vi "2 ‚crans.vi"() -> ()   [LabVIEW 2013]
uses:
  <vilib>/Instr/_visa.llb/VISA Configure Serial Port (Instr).vi
panel:
  out "Distance du drone à la caméra":dbl format="%#_4g"
  out "Taille 2":u32
  out "Taille 1":u32
  out "Taille 4":u32
  out "Taille 3":u32
  out "Y3":u32
  out "X3":u32
  out "Y":u32
  out "X":u32
  out "Y":u32
  out "X1":u32
  out "Y":u32
  out "X":u32
  in  "Y max":i32
  in  "X max":i32
  in  "Y min":i32
  in  "X min":i32
  out "new picture en sortie 2":picture caption="Camera 2"
  out "Chaîne":string
  in  "Attente (ms)":u32=80
  out "new picture en sortie":picture caption="Camera 1"
  out "Chaîne vide":bool
  out "Intrusion dans la\nzone de sécurité !":bool
  out "bytes read":u32
  in  "Source":refnum<visa-resource-name>="COM1"
  in  "stop":bool
  in  "Play":bool
  in  "path to BMP file":path
  # "Ce programme est conçu pour repérer la position des quatre drones ou moins dans une zone a surveiller.\n\nLorsque que l'un des drones rentre dans la zone de haute sécurité ( zone grisée ) une alarme se déclanche, \nen effet, la LED est verte si aucun drone n'est repéré dans la cette zone et elle est rouge si un drone est\ndétecté.\n\nLe programme nous donne aussi la position des drones. Ces informations sont transmises via Wi-Fi grâce à un module X-Bee connecté a un port USB."
  # "La LED de couleur verte indique que les\ndonnées sont en cours de traitement. \nLa LED de couleur rouge indique que le \nprogramme attend les données."
  # "ATTENTION !\nVeillez à ce que la souce de donnée soit\nbranchée sur le port ci-contre.\nSi le port USB correspondant ne s'affiche\npas cliquez sur Rafraichir puis sélectionner \nbon port."
  # "Ce voyant reste vert quand aucun drone ne se trouve dans la zone de sécurité.\nCe voyant s'allume en rouge lorsqu'un drone rentre dans la zone de sécurité.\n\nUn signal sonore est également émis lorsqu'un drone entre dans la zone."
  # "Play / Pause"
  # "Arrêter le programme"
  # "Coordonnées de\nla zone de sécurité"
  # "drone violet"
  # "drone violet"
  # "Position"
  # "Position"
  # "Taille"
  # "Taille"
  # "drone jaune"
  # "drone jaune"
  # "Position"
  # "Position"
  # "Taille"
  # "Taille"
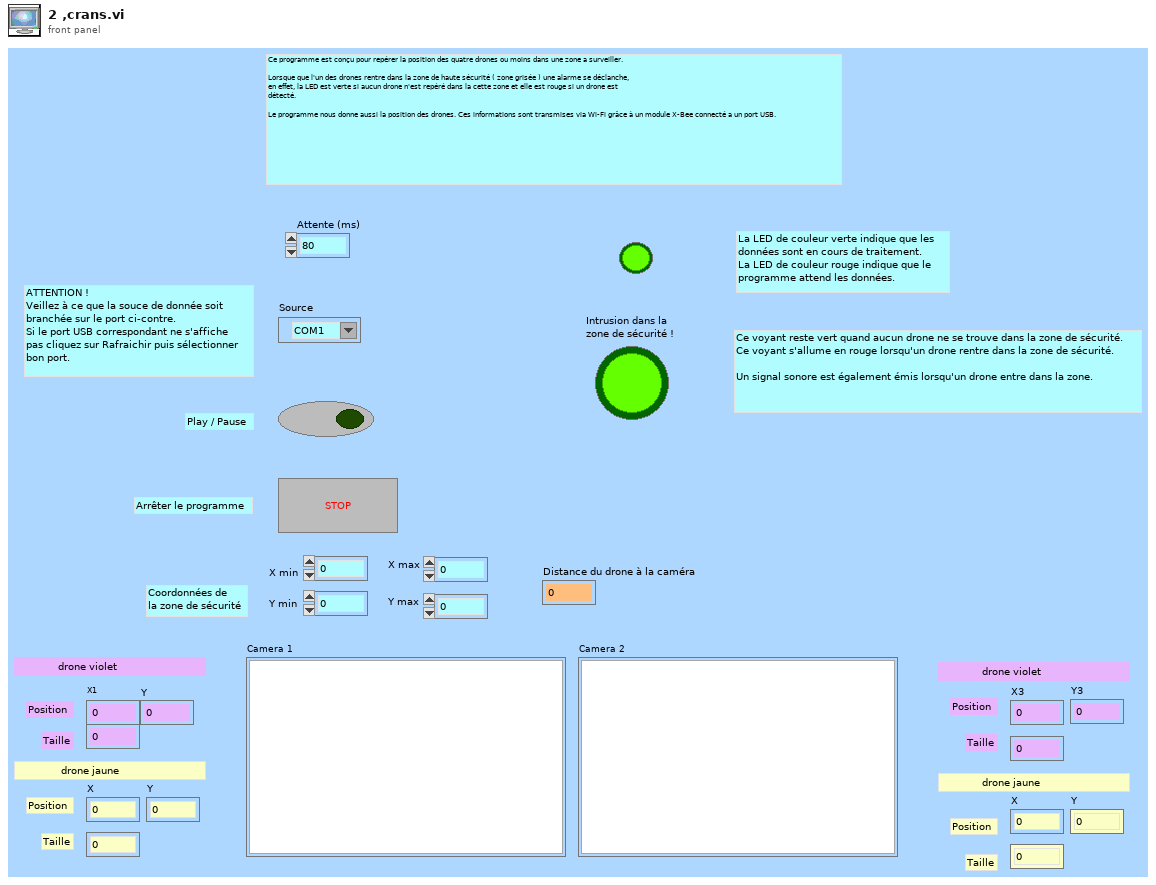
[diagram p1: front panel]
types:
  T1 = typedef "imagedata.ctl" = cluster{"image type":i32, "image depth":i32, "image":u8[], "mask":u8[], "colors":u32[], "Rectangle":cluster{"left":i16, "top":i16, "right":i16, "bottom":i16}}
  T2 = enum32{"Solid", "Dash", "Dot", "DashDot", "DashDotDot"}
  T3 = cluster{cluster{u32, cluster{u32, u32}}, cluster{u32, cluster{u32, u32}}, cluster{u32, cluster{u32, u32}}, cluster{u32, cluster{u32, u32}}}
  T4 = cluster{"S1":cluster{"X (S2;b1) ":u32, "Y (S2;b1)":u32}, "S2":cluster{"X (S2;b1) ":u32, "Y (S2;b1)":u32}, "S3":cluster{"X (S2;b1) ":u32, "Y (S2;b1)":u32}, "S4":cluster{"X (S2;b1) ":u32, "Y (S2;b1)":u32}, "taille (S1)":u32, "taille (S2)":u32, "taille (S3)":u32, "taille (S4)":u32}
  T5 = cluster{cluster{"taille (S1)":u32, "S1":cluster{"X (S2;b1) ":u32, "Y (S2;b1)":u32}}, cluster{"taille (S2)":u32, "S2":cluster{"X (S2;b1) ":u32, "Y (S2;b1)":u32}}, cluster{"taille (S3)":u32, "S3":cluster{"X (S2;b1) ":u32, "Y (S2;b1)":u32}}, cluster{"taille (S4)":u32, "S4":cluster{"X (S2;b1) ":u32, "Y (S2;b1)":u32}}}
  T6 = cluster{"S1":cluster{"X (S1;b1)":u32, "Y (S1;b1)":u32}, "S2":cluster{"X (S1;b2) ":u32, "Y (S1;b2)":u32}, "S3":cluster{"X (S2;b1) ":u32, "Y (S2;b1)":u32}, "S4":cluster{"X (S2;b2)":u32, "Y (S2;b2)":u32}}
  T7 = cluster{"X min":i32, "Y min":i32, "X max":i32, "Y max":i32}
  T8 = cluster{"taille (S1)":u32, "Style":enum32{"Solid", "Dash", "Dot", "DashDot", "DashDotDot"}}
  T9 = cluster{"taille (S3)":u32, "Style":enum32{"Solid", "Dash", "Dot", "DashDot", "DashDotDot"}}
  T10 = cluster{"taille (S4)":u32, "Style":enum32{"Solid", "Dash", "Dot", "DashDot", "DashDotDot"}}
  T11 = cluster{"taille (S2)":u32, "Style":enum32{"Solid", "Dash", "Dot", "DashDot", "DashDotDot"}}
  T12 = cluster{"taille (S1)":u32, "S1":cluster{"X (S2;b1) ":u32, "Y (S2;b1)":u32}}
  T13 = cluster{"taille (S2)":u32, "S2":cluster{"X (S2;b1) ":u32, "Y (S2;b1)":u32}}
  T14 = cluster{"taille (S3)":u32, "S3":cluster{"X (S2;b1) ":u32, "Y (S2;b1)":u32}}
  T15 = cluster{"taille (S4)":u32, "S4":cluster{"X (S2;b1) ":u32, "Y (S2;b1)":u32}}
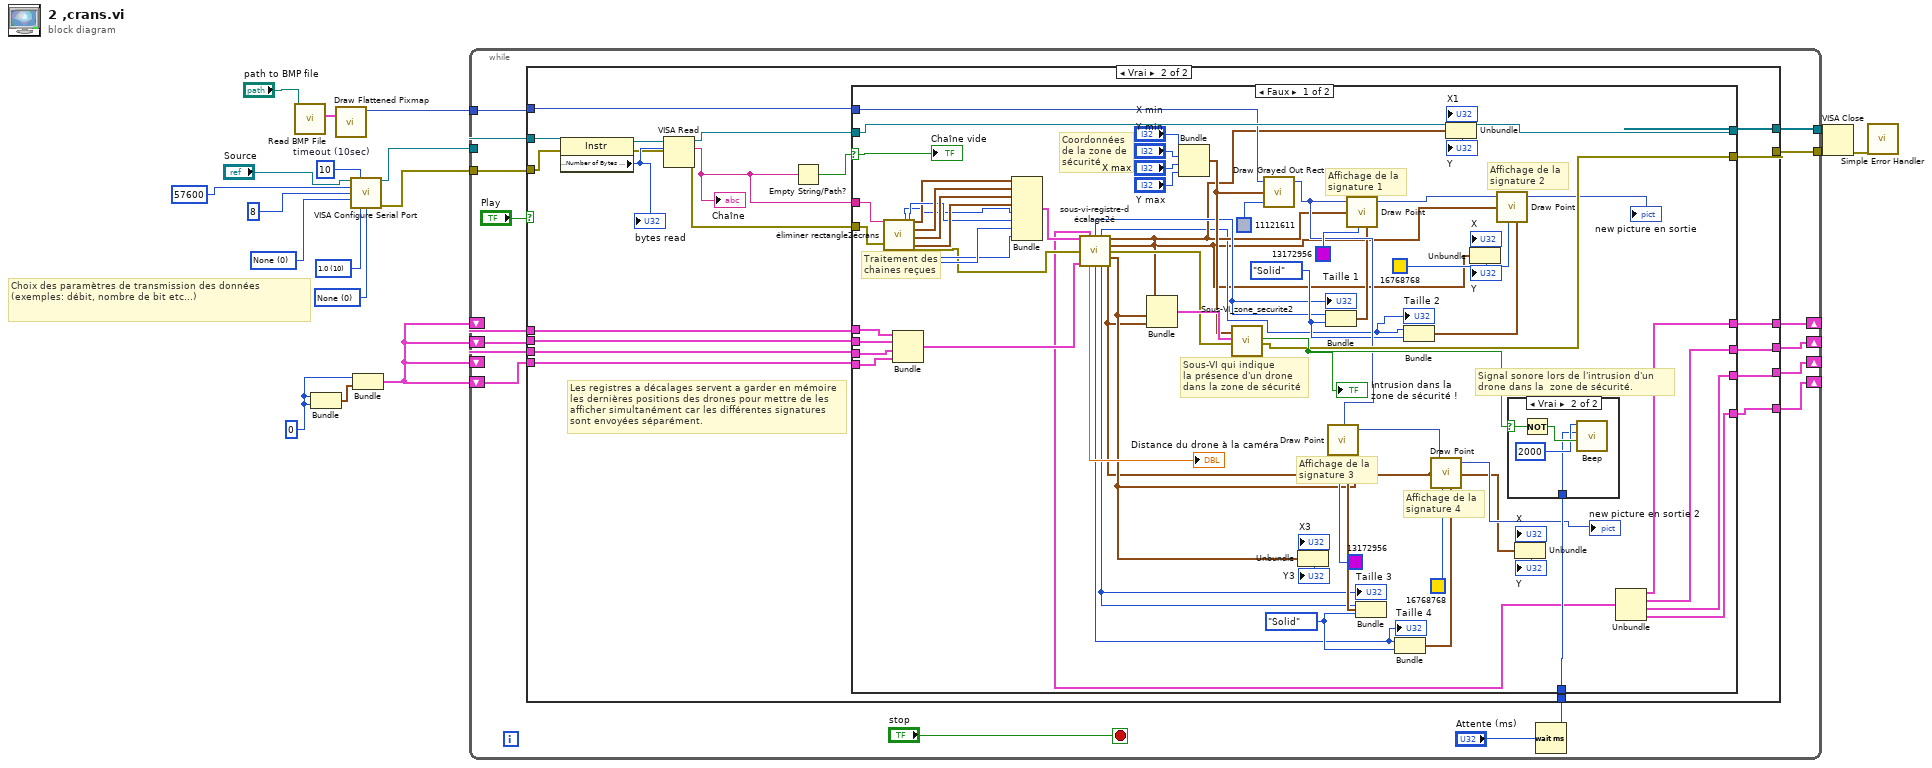
[diagram p0: block diagram]
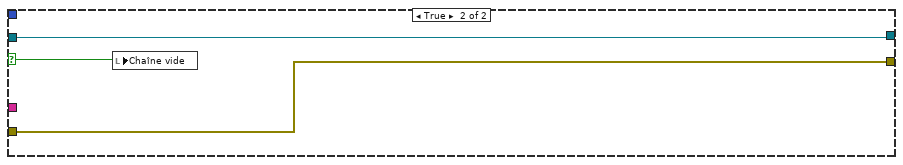
[diagram p4: hidden frame]
diagram:
  w1 = u32 0
  w8 = u16 0 items=["None", "Odd", "Even", "Mark", "Space"] ("parity")
  w10 = u16 10 items=["1.0"=10, "1.5"=15, "2.0"=20] ("stop bits")
  w11 = u16 0 items=["None"=0, "XON/XOFF"=1, "RTS/CTS"=2, "DTR/DSR"=4] ("flow control")
  w9 = u32 10  # timeout (10sec)
  # "Choix des paramètres de transmission des données (exemples: débit, nombre de bit etc...)"
  n1 = call <vilib>:"Read BMP File.vi"("path to BMP file"="path to BMP file") -> ("image data"=w14:T1)  [unwired: 8 in, 2 out]
  n2 = Bundle(w1, w1) -> (w2:cluster{u32, u32})  [unwired: 1 in]
  n3 = call <vilib>:"Draw Flattened Pixmap.vi"("image data"=w14) -> ("new picture"=w13:picture)  [unwired: 8 in]
  n4 = call-poly "VISA Configure Serial Port"("VISA resource name"="Source", "timeout (10sec)"=w9, "baud rate (9600)"=u32 57600 ("baud rate"), "data bits (8)"=u16 8 ("data bits"), "parity (0:none)"=w8, "stop bits (10: 1 bit)"=w10, "flow control (0:none)"=w11) -> ("VISA resource name out"=w5:refnum<visa-resource-name>, "error out"=w4:errorcluster)  [unwired: 7 in]
  n5 = Bundle(w1, w2) -> (w3:cluster{u32, cluster{u32, u32}})  [unwired: 1 in]
  n6 = while {
    tunnel: [w34] -> w17
    tunnel: [w33] -> w16
    tunnel: w13 -> [w32]
    tunnel: w5 -> [w29]
    tunnel: w4 -> [w28]
    shift-right: [w21] -> _
    shift-left: w3 -> [w25]
    shift-right: [w20] -> _
    shift-left: w3 -> [w24]
    shift-right: [w22] -> _
    shift-left: w3 -> [w26]
    shift-right: [w19] -> _
    shift-left: w3 -> [w23]
    stop <- "stop" stop-if-true
    n7 = case shown="Vrai" "Play" {
      tunnel: [w36 w50] -> w34
      tunnel: [w35 w48] -> w33
      tunnel: w32 -> [_ w49]
      tunnel: w29 -> [w36 w51]
      tunnel: w28 -> [w35 w52]
      tunnel: "Attente (ms)" -> [_ w47]
      tunnel: w26 -> [_ w44]
      tunnel: w25 -> [_ w43]
      tunnel: w24 -> [_ w42]
      tunnel: w23 -> [_ w41]
      tunnel: [_ w40] -> w22
      tunnel: [_ w39] -> w21
      tunnel: [_ w38] -> w20
      tunnel: [_ w37] -> w19
      frame False {
      }
      frame True {
        # "Les registres a décalages servent a garder en mémoire\nles dernières positions des drones pour mettre de les\nafficher simultanément car les différentes signatures \nsont envoyées séparément."
        n8 = property class="Instr"(reference=w51, error in=w52) -> (reference out=w57:refnum<visa-resource-name>, error out=w55:errorcluster, "Serial Settings:Number of Bytes at Serial Port"=w56:u32)
        "bytes read" <- w56
        n9 = VISA Read(VISA resource name=w57, byte count=w56, error in (no error)=w55) -> (VISA resource name out=w54:refnum<visa-resource-name>, read buffer=w46:string, error out=w45:errorcluster)  [unwired: 1 out]
        "Chaîne" <- w46
        n10 = Empty String/Path?(string/path=w46) -> (empty?=w53:bool)
        n11 = case shown="Faux" w53 {
          selector: w53 -> [w124 w131]
          tunnel: w54 -> [w125 w132]
          tunnel: [w125 w132] -> w50
          tunnel: w49 -> [w114 _]
          tunnel: [w118 w130] -> w48
          tunnel: w47 -> [w121 _]
          tunnel: w46 -> [w117 _]
          tunnel: w45 -> [w96 w130]
          tunnel: w44 -> [w88 _]
          tunnel: w43 -> [w87 _]
          tunnel: w42 -> [w86 _]
          tunnel: w41 -> [w85 _]
          tunnel: [w62 _] -> w40
          tunnel: [w61 _] -> w39
          tunnel: [w60 _] -> w38
          tunnel: [w59 _] -> w37
          frame False {
            w98 = T2."Solid" ("Style")
            w113 = T2."Solid" ("Style")
            # "Affichage de la\nsignature 4"
            # "Affichage de la\nsignature 3"
            # "Affichage de la\nsignature 2"
            # "Affichage de la\nsignature 1"
            # "Signal sonore lors de l'intrusion d'un \ndrone dans la  zone de sécurité."
            # "Traitement des\nchaines reçues"
            # "Coordonnées\nde la zone de\nsécurité"
            # "Sous-VI qui indique\nla présence d'un drone\ndans la zone de sécurité"
            n12 = call "éliminer rectangle2écrans.vi"("Chaine d'entrée"=w117, "entrée d'erreur (pas d'erreur)"=w96) -> ("taille (S1)"=w58:u32, "taille (S3)"=w91:u32, "taille (S2)"=w92:u32, "taille (S4)"=w90:u32, "S1"=w89:cluster{"X (S2;b1) ":u32, "Y (S2;b1)":u32}, "S2"=w95:cluster{"X (S2;b1) ":u32, "Y (S2;b1)":u32}, "S3"=w94:cluster{"X (S2;b1) ":u32, "Y (S2;b1)":u32}, "S4"=w93:cluster{"X (S2;b1) ":u32, "Y (S2;b1)":u32}, "sortie d'erreur"=w83:errorcluster)  [unwired: 17 in]
            n13 = Bundle(w88, w87, w86, w85) -> (w72:T3)  [unwired: 1 in]
            n14 = Bundle("S1"=w89, "S2"=w95, "S3"=w94, "S4"=w93, "taille (S1)"=w58, "taille (S2)"=w92, "taille (S3)"=w91, "taille (S4)"=w90) -> (w84:T4)  [unwired: 1 in]
            n15 = call "sous-vi-registre-décalage2é.vi"("Cluster traitement"=w84, "entrée erreur"=w83, "Cluster"=w72) -> ("Cluster en sortie"=w63:T5, "taille (S1)"=w71:u32, "taille (S2)"=w69:u32, "S1"=w70:cluster{"X (S1;b1)":u32, "Y (S1;b1)":u32}, "S2"=w68:cluster{"X (S1;b2) ":u32, "Y (S1;b2)":u32}, "constante d'erreur"=w82:errorcluster, "S3"=w66:cluster{"X (S2;b1) ":u32, "Y (S2;b1)":u32}, "Distance entre la caméra et le drone"=→"Distance du drone à la caméra":dbl, "taille (S4)"=w65:u32, "taille (S3)"=w67:u32, "S4"=w64:cluster{"X (S2;b2)":u32, "Y (S2;b2)":u32})  [unwired: 2 in]
            "Taille 3" <- w67
            "Taille 4" <- w65
            "Taille 1" <- w71
            "Taille 2" <- w69
            n16 = Bundle("S1"=w70, "S2"=w68, "S3"=w66, "S4"=w64) -> (w120:T6)  [unwired: 1 in]
            n17 = Bundle("X min"="X min", "Y min"="Y min", "X max"="X max", "Y max"="Y max") -> (w104:T7)  [unwired: 1 in]
            n18 = call "Sous-VI_zone_securite2.vi"("Coordonnées des drônes"=w120, "constante ii 2"=w82, "Coordonnées du rectangle"=w104) -> ("Booléen"=w119:bool, "constante d'erreur"=w118:errorcluster)  [unwired: 15 in]
            "Intrusion dans la\nzone de sécurité !" <- w119
            n19 = call <vilib>:"Draw Grayed Out Rect.vi"("color(black)"=u32 11121611, "rect"=w104, "picture"=w114) -> ("new picture"=w112:picture)  [unwired: 2 in]
            n20 = Unbundle(w66) -> ("X (S2;b1)"=→"X3":u32, "Y (S2;b1)"=→"Y3":u32)
            n21 = Bundle ("S1")("taille (S1)"=w71, "Style"=w98) -> (w103:T8)  [unwired: 1 in]
            n22 = call <vilib>:"Draw Point.vi"("picture"=w112, "point(x,y)"=w70, "color(black)"=u32 13172956, "pen"=w103) -> ("new picture"=w116:picture)  [unwired: 5 in]
            n23 = Bundle ("S3")("taille (S3)"=w67, "Style"=w113) -> (w99:T9)  [unwired: 1 in]
            n24 = call <vilib>:"Draw Point.vi"("picture"=w112, "point(x,y)"=w66, "color(black)"=u32 13172956, "pen"=w99) -> ("new picture"=w111:picture)  [unwired: 5 in]
            n25 = Bundle ("S4")("taille (S4)"=w65, "Style"=w113) -> (w100:T10)  [unwired: 1 in]
            n26 = Bundle ("S2")("taille (S2)"=w69, "Style"=w98) -> (w97:T11)  [unwired: 1 in]
            n27 = call <vilib>:"Draw Point.vi"("picture"=w111, "point(x,y)"=w64, "color(black)"=u32 16768768, "pen"=w100) -> ("new picture"=→"new picture en sortie 2":picture)  [unwired: 5 in]
            n28 = Unbundle(w70) -> ("X (S1;b1)"=→"X1":u32, "Y (S1;b1)"=→"Y":u32)
            n29 = Unbundle(w68) -> ("X (S1;b2)"=→"X":u32, "Y (S1;b2)"=→"Y":u32)
            n30 = call <vilib>:"Draw Point.vi"("picture"=w116, "point(x,y)"=w68, "color(black)"=u32 16768768, "pen"=w97) -> ("new picture"=→"new picture en sortie":picture)  [unwired: 5 in]
            n31 = case shown="Vrai" w119 {
              selector: w119 -> [_ w129]
              tunnel: w121 -> [_ w126]
              frame False {
              }
              frame True {
                n32 = Not(x=w129) -> (.not. x?=w128:bool)
                n33 = call <vilib>:"Beep.vi"("use system alert? (T)"=w128, "duration (msec)"=w126, "frequency (Hz)"=2000) -> ()  [unwired: 9 in]
              }
            }
            n34 = Unbundle(w64) -> ("X (S2;b2)"=→"X":u32, "Y (S2;b2)"=→"Y":u32)
            n35 = Unbundle(w63) -> (w62:T12, w61:T13, w60:T14, w59:T15)
            "Chaîne vide" <- w124
          }
          frame True {
            n36 = local write "Chaîne vide"(w131) -> ()
          }
        }
      }
    }
    n37 = Wait (ms)(milliseconds to wait="Attente (ms)") -> ()  [unwired: 1 out]
  }
  n38 = VISA Close(VISA resource name=w17, error in (no error)=w16) -> (error out=w18:errorcluster)
  n39 = call <vilib>:"Simple Error Handler.vi"("error in (no error)"=w18) -> ()  [unwired: 4 in, 5 out]
